vi "Mathcad variables.vi"() -> ()   [LabVIEW 2010]
uses:
  <vilib>/Utility/file.llb/Write To Spreadsheet File (string).vi
panel:
  out "Full Names":string[][](array[string])
  in  "Save to XLS":bool
  out "XML":string
  in  "Find Variables":bool
  in  "stop":bool
  in  "Path":path
  # "Select a single file"
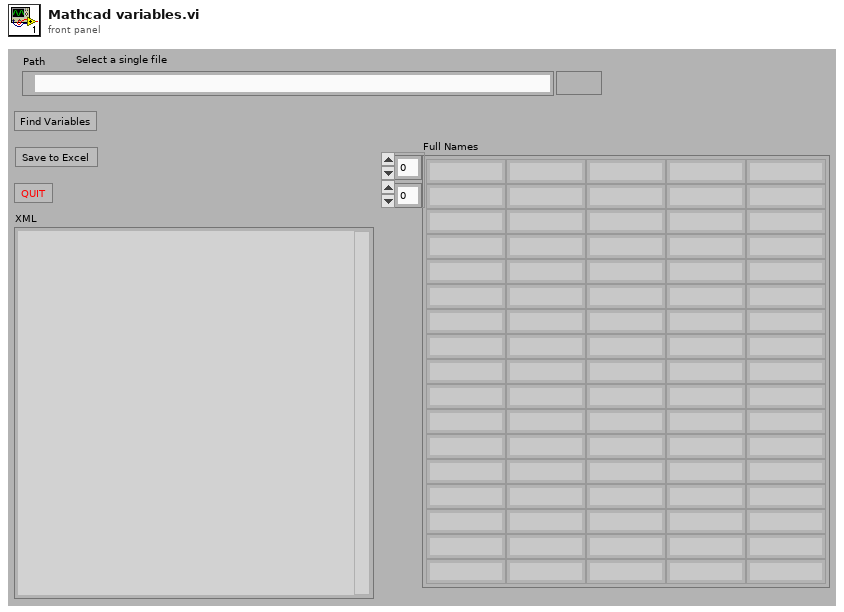
[diagram p1: front panel]
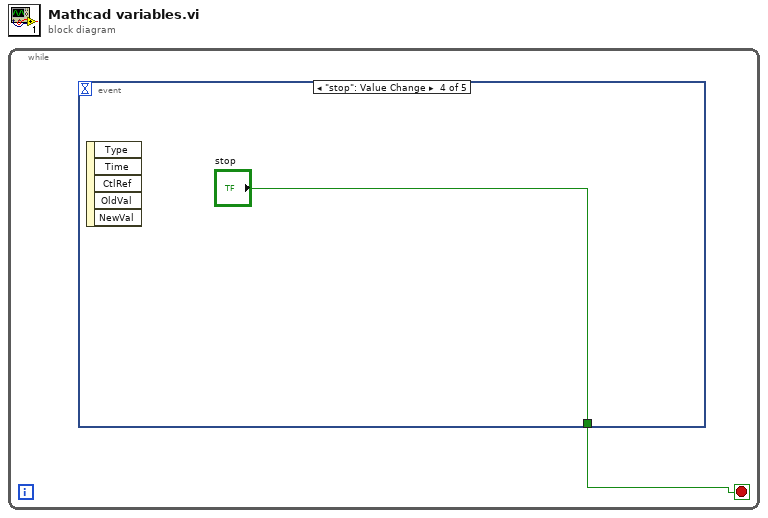
[diagram p0: block diagram]
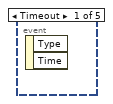
[diagram p2: hidden frame]
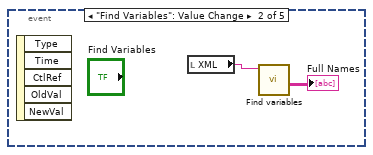
[diagram p3: hidden frame]
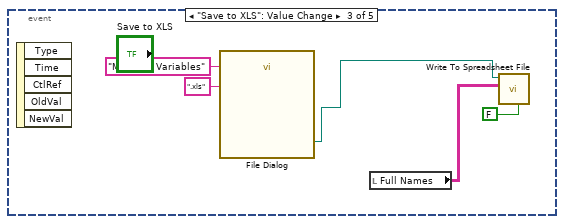
[diagram p4: hidden frame]
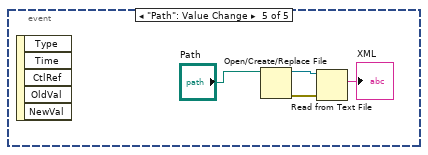
[diagram p5: hidden frame]
diagram:
  n1 = while {
    stop <- w1 stop-if-true
    n2 = event shown="[3] \"stop\": Value Change" {
      selector: _ -> [_ _ _ _ _]
      dyn-events: _ -> [_ _ _ _ _]
      timeout: _ -> [_ _ _ _ _]
      tunnel: [_ _ _ "stop" _] -> w1
      event Timeout {
        n3 = event-data() -> ()  [unwired: 1 in, 2 out]
      }
      event "Find Variables": Value Change {
        n4 = event-data() -> ()  [unwired: 1 in, 5 out]
        n5 = local read "XML"() -> (w3:string)
        n6 = call "Find variables.vi"("XML"=w3) -> ("Full Names"=→"Full Names":string[][])  [unwired: 9 in, 1 out]
      }
      event "Save to XLS": Value Change {
        n7 = event-data() -> ()  [unwired: 1 in, 5 out]
        n8 = call "File Dialog"("default name"="Mathcad Variables", "pattern (all files)"=".xls") -> ("selected path"=w5:path)  [unwired: 10 in, 3 out]
        n9 = local read "Full Names"() -> (w4:string[][])
        n10 = call-poly <vilib>:"Write To Spreadsheet File.vi"("transpose? (no:F)"=FALSE, "2D data"=w4, "file path (dialog if empty)"=w5) -> ()  [unwired: 5 in, 1 out]
      }
      event "stop": Value Change {
        n11 = event-data() -> ()  [unwired: 1 in, 5 out]
      }
      event "Path": Value Change {
        n12 = event-data() -> ()  [unwired: 1 in, 5 out]
        n13 = Open/Create/Replace File(file path (use dialog)="Path") -> (refnum out=w11:refnum<file>, error out=w12:errorcluster)  [unwired: 5 in, 1 out]
        n14 = Read from Text File(file (use dialog)=w11, error in=w12) -> (text=→"XML":string)  [unwired: 2 in, 3 out]
      }
    }
  }
